vi "Add Mode Code.vi"(4 "create timestamp channel":bool, 6 "parameters":T2(array[cluster]), 7 "mode code":u16=1, 8 "error in":errorcluster, 9 "terminals":cluster{"Rx":T3, "Tx":T3}, 10 "name":string, 11 "port in":T5 format="%.0x") -> (0 "error out":errorcluster, 3 "port out":T5 format="%.0x")   [LabVIEW 2020, in "Ballard MIL-STD-1553 Scripting.lvlib"]
uses:
  Ballard MIL-STD-1553 Scripting.lvlib
  <vilib>/NI VeriStand/Custom Device API/Custom Device Item Ref.ctl
  Shared/Terminal Endpoint.ctl
  Shared/Address.ctl
  Shared/Parameter Definition.ctl
  <vilib>/NI VeriStand/Custom Device API/Custom Device API.lvlib
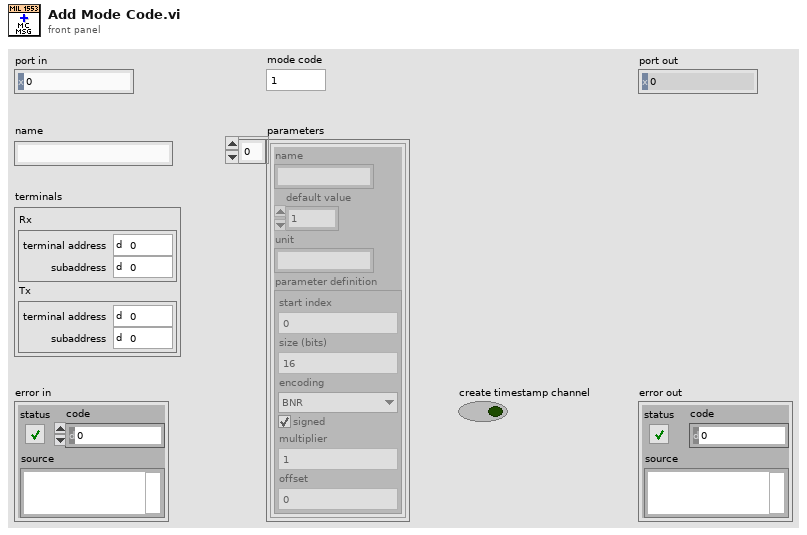
[diagram p1: front panel]
types:
  T1 = typedef "Parameter Definition.ctl" = cluster{"start index":i32, "size (bits)":i32, "encoding":enum16{"BNR", "BCD", "Discrete"}, "signed":bool, "multiplier":dbl, "offset":dbl}
  T2 = cluster{"name":string, "default value":dbl, "unit":string, "parameter definition":T1}[]
  T3 = typedef "Terminal Endpoint.ctl" = cluster{"terminal address":T4, "subaddress":T4}
  T4 = typedef "Address.ctl" = u16
  T5 = typedef "Custom Device API.lvlib/Custom Device Item Ref.ctl" = u64
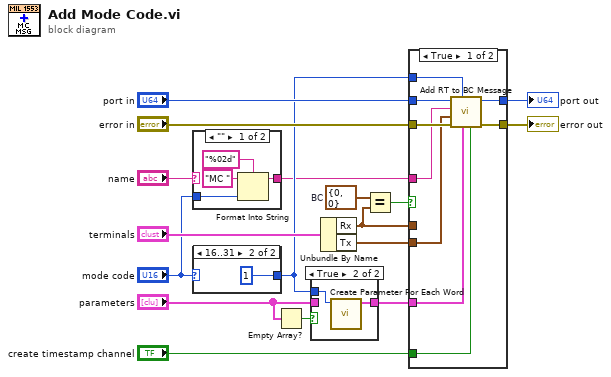
[diagram p0: block diagram]
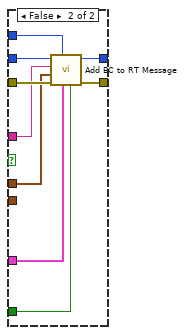
[diagram p3: hidden frame]
diagram:
  w14 = T3 {"terminal address"=0, "subaddress"=0}  # BC
  n1 = case shown="\"\"" "name" {
    selector: "name" -> [_ w22]
    tunnel: [w21 w22] -> w2
    tunnel: "mode code" -> [w19 _]
    frame "" {
      n2 = Format Into String(format string="%02d", initial string="MC ", w19) -> (resulting string=w21:string)  [unwired: 1 in, 1 out]
    }
    frame Default {
    }
  }
  n3 = case shown="16..31" "mode code" {
    tunnel: [_ u16 1 ("mode code")] -> w5
    frame Default {
    }
    frame 16..31 {
    }
  }
  n4 = Empty Array?(array="parameters") -> (empty?=w17:bool)
  n5 = case shown="True" w17 {
    tunnel: w5 -> [_ w26]
    tunnel: "parameters" -> [w24 _]
    tunnel: [w24 w25] -> w8
    frame False {
    }
    frame True {
      n6 = call "Create Parameter For Each Word.vi"("number of words"=w26) -> ("parameters"=w25:T2)  [unwired: 9 in, 1 out]
    }
  }
  n7 = Unbundle By Name("terminals") -> ("Rx"=w4:T3, "Tx"=w6:T3)
  n8 = Equal?(x=w14, y=w4) -> (x = y?=w13:bool)
  n9 = case shown="True" w13 {
    tunnel: "port in" -> [w35 w44]
    tunnel: "error in" -> [w34 w43]
    tunnel: [w33 w42] -> w10
    tunnel: [w32 w41] -> w9
    tunnel: w8 -> [w31 w40]
    tunnel: "create timestamp channel" -> [w30 w39]
    tunnel: w2 -> [w29 w38]
    tunnel: w6 -> [w28 _]
    tunnel: w5 -> [w27 w37]
    tunnel: w4 -> [_ w36]
    frame True {
      n10 = call "Add RT to BC Message.vi"("create timestamp channel"=w30, "parameters"=w31, "number of words"=w27, "error in"=w34, "Tx remote terminal"=w28, "name"=w29, "port in"=w35) -> ("error out"=w33:errorcluster, "port out"=w32:T5)  [unwired: 3 in]
    }
    frame False {
      n11 = call "Add BC to RT Message.vi"("create timestamp channel"=w39, "parameters"=w40, "number of words"=w37, "error in"=w43, "Rx remote terminal"=w36, "name"=w38, "port in"=w44) -> ("error out"=w42:errorcluster, "port out"=w41:T5)  [unwired: 3 in]
    }
  }
  "error out" <- w10
  "port out" <- w9
